vi "CheckLoopFinish.vi"(7 "Deviation":bool, 8 "error in":errorcluster, 9 "maxRuns":i32=10, 10 "iCounter":i32, 11 "Frequency List":T1(array[cluster])) -> (3 "Stop Loop":bool, 5 "maxRuns":bool)   [LabVIEW 2018]
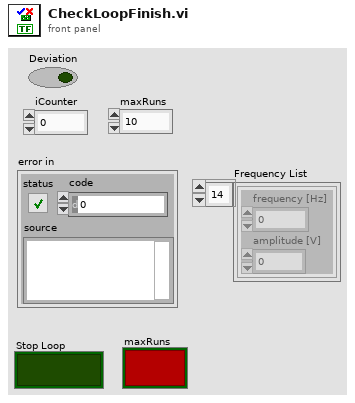
[diagram p1: front panel]
types:
  T1 = cluster{"frequency [Hz]":dbl, "amplitude [V]":dbl}[]
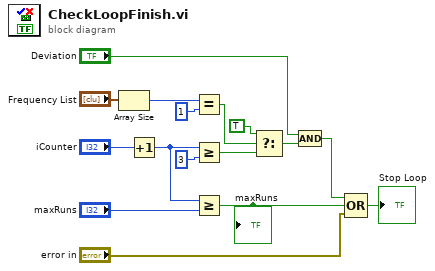
[diagram p0: block diagram]
diagram:
  n1 = Array Size(array="Frequency List") -> (size(s)=w5:i32)
  n2 = Increment(x="iCounter") -> (x+1=w4:i32)
  n3 = Equal?(x=w5, y=1) -> (x = y?=w15:bool)
  n4 = Greater Or Equal?(x=w4, y=3) -> (x >= y?=w9:bool)
  n5 = Greater Or Equal?(x=w4, y="maxRuns") -> (x >= y?=w2:bool)
  "maxRuns" <- w2
  n6 = Select(t=TRUE, s=w15, f=w9) -> (s? t:f=w11:bool)
  n7 = Compound Arithmetic op=AND("Deviation", w11) -> (w7:bool)
  n8 = Compound Arithmetic op=OR(w7, w2, "error in") -> (→"Stop Loop":bool)
